vi "Data Min-Max.vi"(0 "VISA resource name":refnum<visa-resource-name>, 7 "Input (1)":dbl=1.0 min=1.0 max=8.0 step=1.0, 11 "error in (no error)":errorcluster) -> (4 "VISA resource name out":refnum<visa-resource-name>, 6 "Min Reading":dbl min=-9999.9 max=9999.9 step=0.0001 format="%.4f", 8 "Max Reading":dbl min=-9999.9 max=9999.9 step=0.0001 format="%.4f", 15 "error out":errorcluster)   [LabVIEW 2017, in "Lake Shore Cryotronics 218.lvlib"]
doc: "This VI reads the min/max data for a selected input. Data read will be in the format selected with the Math function. See the Config. Math.VI for more information."
uses:
  Lake Shore Cryotronics 218.lvlib
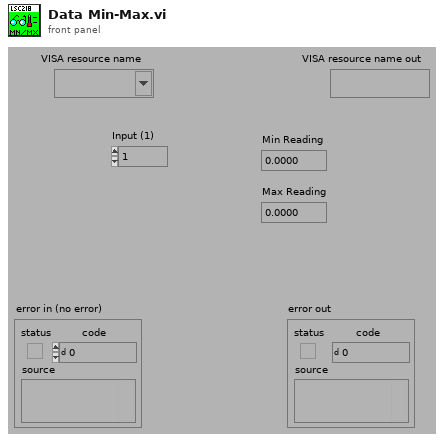
[diagram p1: front panel]
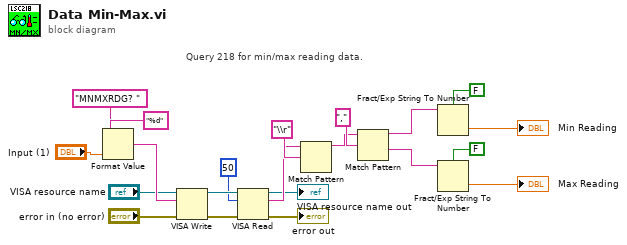
[diagram p0: block diagram]
diagram:
  # "Query 218 for min/max reading data."
  n1 = Format Value(string ("")="MNMXRDG? ", format string="%d", value (0)="Input (1)") -> (output string=w13:string)
  n2 = VISA Write(VISA resource name="VISA resource name", write buffer=w13, error in (no error)="error in (no error)") -> (VISA resource name out=w21:refnum<visa-resource-name>, error out=w20:errorcluster)  [unwired: 1 out]
  n3 = VISA Read(VISA resource name=w21, byte count=50, error in (no error)=w20) -> (VISA resource name out=→"VISA resource name out":refnum<visa-resource-name>, read buffer=w18:string, error out=→"error out":errorcluster)  [unwired: 1 out]
  n4 = Match Pattern(string=w18, regular expression="\\r") -> (before substring=w10:string)  [unwired: 1 in, 3 out]
  n5 = Match Pattern(string=w10, regular expression=",") -> (before substring=w12:string, after substring=w8:string)  [unwired: 1 in, 2 out]
  n6 = Fract/Exp String To Number(use system decimal point (T)=FALSE, string=w12) -> (number=→"Min Reading":dbl)  [unwired: 2 in, 1 out]
  n7 = Fract/Exp String To Number(use system decimal point (T)=FALSE, string=w8) -> (number=→"Max Reading":dbl)  [unwired: 2 in, 1 out]
